vi "Spectral Map (Analog Tach).vi"(4 "window info":T4={"window type"=3, "window length"=2048} {"window type" items=["None"=0, "Hanning"=1, "Hamming"=2, "Blackman-Harris"=3, "Exact Blackman"=4, "Blackman"=5, "Flat Top"=6, "4 Term B-Harris"=7, "7 Term B-Harris"=8, "Low Sidelobe"=9, "Gaussian"=62]; "window length" min=0}, 6 "type":T5(ring)=enum."RPM-Order", 7 "dB On (T)":bool=TRUE, 8 "pulse/revolution (1)":dbl=1.0 format="%.2f", 9 "analog tach signal":waveform(dbl)={"t0"=timestamp(0 s since 1904-01-01), "dt"=0.0, "Y"=[]}, 11 "scaled signal [EU]":waveform(dbl)={"t0"=timestamp(0 s since 1904-01-01), "dt"=0.0, "Y"=[]}) -> (0 "speed profile":T1 {"speed [RPM]" format="%.2f"; "time [s]" format="%.2f"}, 1 "unit labels":T2, 2 "scales":T3 {"Y scale"."multiplier" format="%.2f"; "Y scale"."offset" format="%.2f"; "X scale"."multiplier" format="%.2f"; "X scale"."offset" format="%.2f"}, 3 "spectral map":dbl[][](array[numeric]) format="%.2f")   [LabVIEW 2017]
doc: "Returns the spectral map of <B>scaled signal </B>using <B>analog tach signal</B>. You can specify the spectral map type as frequency-time, frequency-RPM, order-RPM, or RPM-order."
uses:
  <vilib>/addons/Sound and Vibration/Order Analysis/Ref Gabor Order Tracking/window information.ctl
  <vilib>/addons/Sound and Vibration/Order Analysis/Tach Process/SubVIs/speed profile.ctl
  <vilib>/addons/Sound and Vibration/Order Analysis/Backward Compatibility/Get Spectral Map (DBL).vi
  <vilib>/addons/Sound and Vibration/Order Analysis/Tach Process/SoundVib_TachProcess.lvlib
  <vilib>/addons/Sound and Vibration/Order Analysis/Gabor Order Tracking/SoundVib_Gabor.lvlib
panel:
  # "Spectral Map (Analog Tach)"
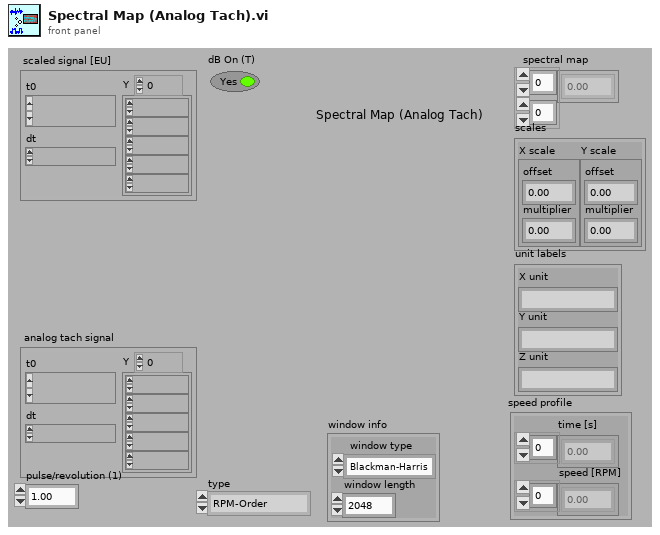
[diagram p1: front panel]
types:
  T1 = typedef "SoundVib_TachProcess.lvlib/speed profile.ctl" = cluster{"time [s]":dbl[], "speed [RPM]":dbl[]}
  T2 = cluster{"X unit":string, "Y unit":string, "Z unit":string}
  T3 = cluster{"X scale":cluster{"offset":dbl, "multiplier":dbl}, "Y scale":cluster{"offset":dbl, "multiplier":dbl}}
  T4 = typedef "SoundVib_Gabor.lvlib/window information.ctl" = cluster{"window type":u32, "window length":i32}
  T5 = enum16{"Frequency-Time", "Frequency-RPM", "Order-RPM", "RPM-Order"}
  T6 = cluster{"X scale":cluster{"offset":dbl, "multiplier":dbl}, "Y scale":cluster{"offset":dbl, "multiplier":dbl}, "Z scale":cluster{"offset":dbl, "multiplier":dbl}}
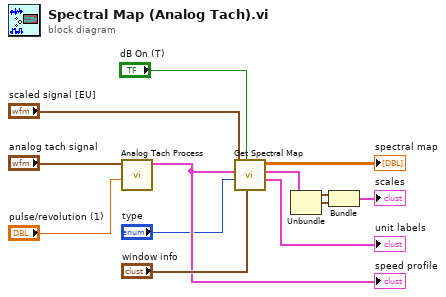
[diagram p0: block diagram]
diagram:
  n1 = call <vilib>:"Analog Tach Process.vi"("pulse/revolution (1)"="pulse/revolution (1)", "analog tach signal"="analog tach signal") -> ("speed profile"=w7:T1)  [unwired: 7 in, 2 out]
  "speed profile" <- w7
  n2 = call-poly <vilib>:"Get Spectral Map.vi"("window info"="window info", "dB On (T)"="dB On (T)", "type"="type", "speed profile"=w7, "scaled signal [EU]"="scaled signal [EU]") -> ("unit labels"=→"unit labels":T2, "scales"=w6:T6, "spectral map"=→"spectral map":dbl[][])  [unwired: 2 in, 2 out]
  n3 = Unbundle(w6) -> ("X scale"=w5:cluster{"offset":dbl, "multiplier":dbl}, "Y scale"=w4:cluster{"offset":dbl, "multiplier":dbl})  [unwired: 1 out]
  n4 = Bundle("X scale"=w5, "Y scale"=w4) -> (→"scales":T3)  [unwired: 1 in]
